vi "GetAttributeByName.vi"(8 "error in (no error)":errorcluster, 10 "AttrName":string, 11 "SMO in":refnum<class "SMO.lvclass">) -> (0 "error out":errorcluster, 1 "found":bool, 2 "Attribute":refnum<class "Attribute.lvclass">, 3 "SMO out":refnum<class "SMO.lvclass">)   [LabVIEW 2021, in "smo.lvlib" / "SMO.lvclass"]
uses:
  SMO.lvclass
  SMO.lvclass/SMO.ctl
  Support/Attribute/Attribute.lvclass
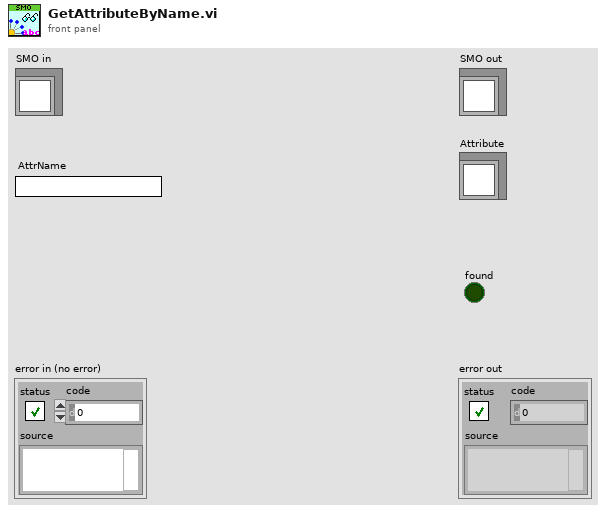
[diagram p1: front panel]
types:
  T1 = typedef "smo.lvlib/def.SMO.lvclass/Scope -- Enum.ctl" = enum16{"Public", "Protected", "Private"}
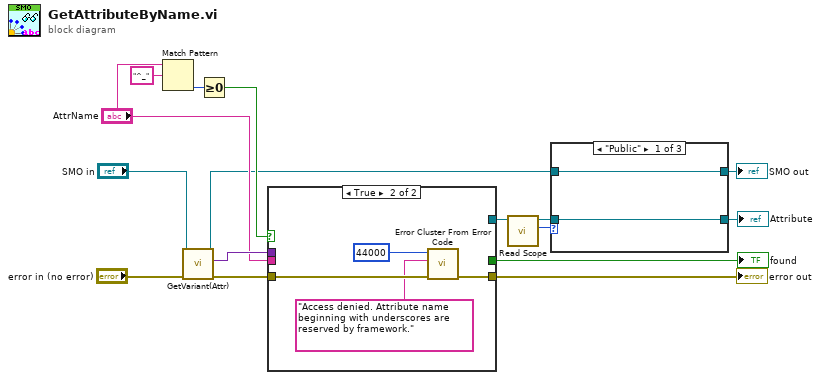
[diagram p0: block diagram]
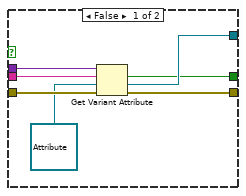
[diagram p4: hidden frame]
diagram:
  n1 = Match Pattern(string="AttrName", regular expression="^_") -> (offset past match=w8:i32)  [unwired: 1 in, 3 out]
  n2 = call "GetVariant(Attr).vi"("error in (no error)"="error in (no error)", "SMO in"="SMO in") -> ("error out"=w14:errorcluster, "[Attributes]"=w12:variant, "SMO out"=w5:refnum<class "SMO.lvclass">)  [unwired: 7 in]
  n3 = Greater Or Equal To 0?(x=w8) -> (x >= 0?=w7:bool)
  n4 = case shown="True" w7 {
    tunnel: w14 -> [w23 w26]
    tunnel: [w22 w27] -> w13
    tunnel: w12 -> [w20 _]
    tunnel: [w19 _] -> w3
    tunnel: [w18 _] -> w11
    tunnel: "AttrName" -> [w17 _]
    frame False {
      n5 = Get Variant Attribute(Variant=w20, name=w17, default value (empty Variant)=refnum<class "Attribute.lvclass"> refnum ("Attribute.lvclass"), error in=w23) -> (found=w18:bool, value=w19:refnum<class "Attribute.lvclass">, error out=w22:errorcluster)  [unwired: 1 out]
    }
    frame True {
      n6 = call <vilib>:"Error Cluster From Error Code.vi"("error in (no error)"=w26, "error message (\"\")"="Access denied. Attribute name beginning with underscores are reserved by framework." ("error message (\"\")"), "error code (0)"=44000) -> ("error out"=w27:errorcluster)  [unwired: 6 in]
    }
  }
  "error out" <- w13
  "found" <- w11
  n7 = call "Read Scope.vi"("Attribute in"=w3) -> ("Scope"=w2:T1, "Attribute out"=w1:refnum<class "Attribute.lvclass">)  [unwired: 9 in]
  n8 = case shown="\"Public\"" w2 {
    tunnel: [w29 w31 w33] -> w6
    tunnel: w5 -> [w29 w31 w33]
    tunnel: [w28 w30 w32] -> w4
    tunnel: w1 -> [w28 w30 w32]
    frame "Public" {
    }
    frame "Protected" {
    }
    frame "Private" {
    }
  }
  "SMO out" <- w6
  "Attribute" <- w4
